vi "rad_Find App Img File.vi"(8 "Error In":errorcluster, 11 "Temp Image Path":path) -> (0 "Error Out":errorcluster, 3 "LVAppImg Path":path)   [LabVIEW 2020]
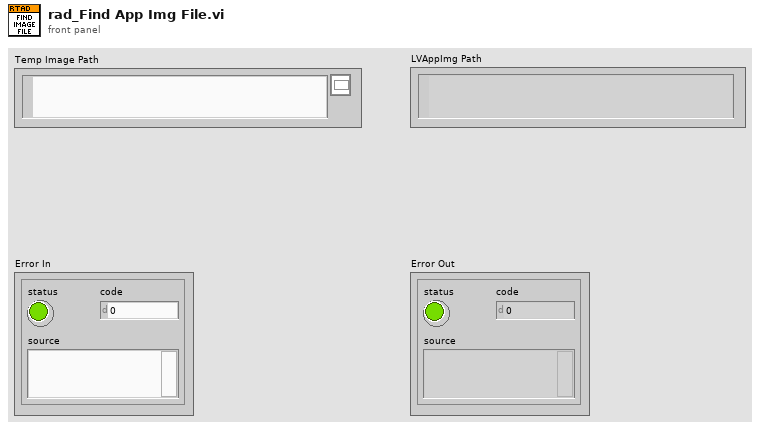
[diagram p1: front panel]
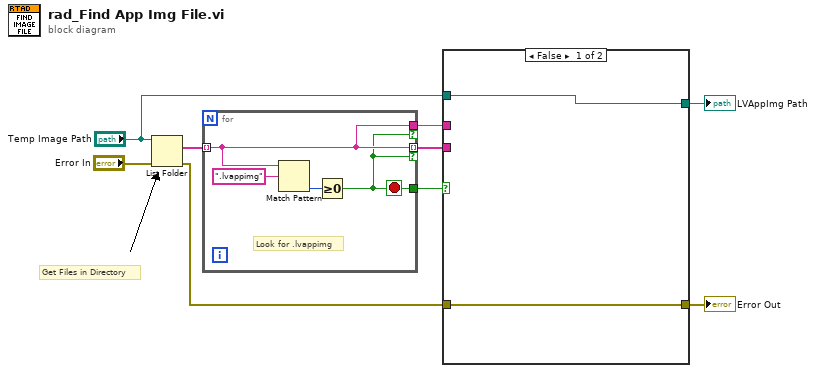
[diagram p0: block diagram]
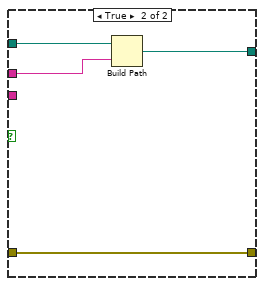
[diagram p2: hidden frame]
diagram:
  # "Get Files in Directory"
  n1 = List Folder(path="Temp Image Path", error in="Error In") -> (filenames=w8:string[], error out=w3:errorcluster)  [unwired: 2 in, 2 out]
  n2 = for {
    tunnel: w8 -> [w12] mode=indexing
    tunnel: [w12] -> w7 mode=indexing if=w10
    tunnel: [w12] -> w4 if=w10
    tunnel: [w10] -> w1
    stop <- w10 stop-if-true
    # "Look for .lvappimg"
    n3 = Match Pattern(string=w12, regular expression=".lvappimg") -> (offset past match=w11:i32)  [unwired: 1 in, 3 out]
    n4 = Greater Or Equal To 0?(x=w11) -> (x >= 0?=w10:bool)
  }
  n5 = case shown="False" w1 {
    tunnel: w7 -> [_ _]
    tunnel: "Temp Image Path" -> [w15 w19]
    tunnel: [w15 w18] -> w5
    tunnel: w4 -> [_ w17]
    tunnel: w3 -> [w14 w16]
    tunnel: [w14 w16] -> w2
    frame False {
    }
    frame True {
      n6 = Build Path(base path=w19, name or relative path=w17) -> (appended path=w18:path)
    }
  }
  "Error Out" <- w2
  "LVAppImg Path" <- w5
